vi "Gaussmeter425_BvsTime.vi"() -> ()   [LabVIEW 2014]
uses:
  <vilib>/Platform/TimedLoop/XDataNode/timing_clust.ctl
  <vilib>/Platform/TimedLoop/XDataNode/nitl_modes.ctl
  <vilib>/Platform/TimedLoop/XDataNode/wakeup.ctl
  <instrlib>/Agilent 3446X Series/Public/Data/Read (Single Point).vi
  <instrlib>/Lake Shore 425/Public/Data/Field Data (Single Reading).vi
  <vilib>/Utility/file.llb/Write To Spreadsheet File (DBL).vi
  <vilib>/Platform/TimedLoop/XDataNode/XDataNode.xnode
  <instrlib>/Lake Shore 425/Lake Shore 425.lvlib
  <vilib>/Platform/TimedLoop/XDataNode/XDNodeRunTimeDep.lvlib
  <instrlib>/Agilent 3446X Series/Agilent 3446X Series.lvlib
panel:
  in  "10 A Mode":bool
  out "Output file name":string
  in  "Use multimeter ON / OFF":bool=TRUE
  in  "Comments":string
  in  "Setup":string(combo)
  out "?":dbl(graph)
  in  "VISA resource name MM":refnum<visa-resource-name>="USB0::0x0957::0x1A07::MY53203201::INSTR"
  in  "Measurement Function (10: Voltage DC)":i32(ring)=10 items=["Current DC"=2, "Voltage DC"=10]
  out "Current [A]":dbl
  out "Magnetic Flux [mT]":dbl
  in  "day":dbl
  in  "h":dbl
  in  "min":dbl
  in  "sec":dbl
  out "Time since run start [s]":dbl
  in  "VISA resource name GM":refnum<visa-resource-name>="COM4"
  in  "Measurements per second:":dbl=1.0
  out "?":dbl(graph)
  in  "?":bool
  in  "Serial Configuration":T1={"Baud Rate"=57600, "Parity"=1, "Data Bits"=7, "Stop Bits"=10, "Flow Control"=0} {"Flow Control" items=["None", "XON/XOFF", "RTS/CTS", "XON/XOFF & RTS/CTS", "DTR/DSR", "XON/XOFF & DTR/DSR"]; "Stop Bits" items=["1.0"=10, "1.5"=15, "2.0"=20]; "Data Bits" items=["7"=7, "8"=8]; "Parity" items=["None", "Odd", "Even", "Mark", "Space"]; "Baud Rate" items=["300"=300, "600"=600, "1200"=1200, "2400"=2400, "4800"=4800, "9600"=9600, "19200"=19200, "38400"=38400, "57600"=57600]}
  # "Automatically stop after..."
  # "more than 3 may not work"
  # "Gaussmeter"
  # "Multimeter"
  # "USB0::0x0957: for multimeter"
  # "Voltage DC for Amp"
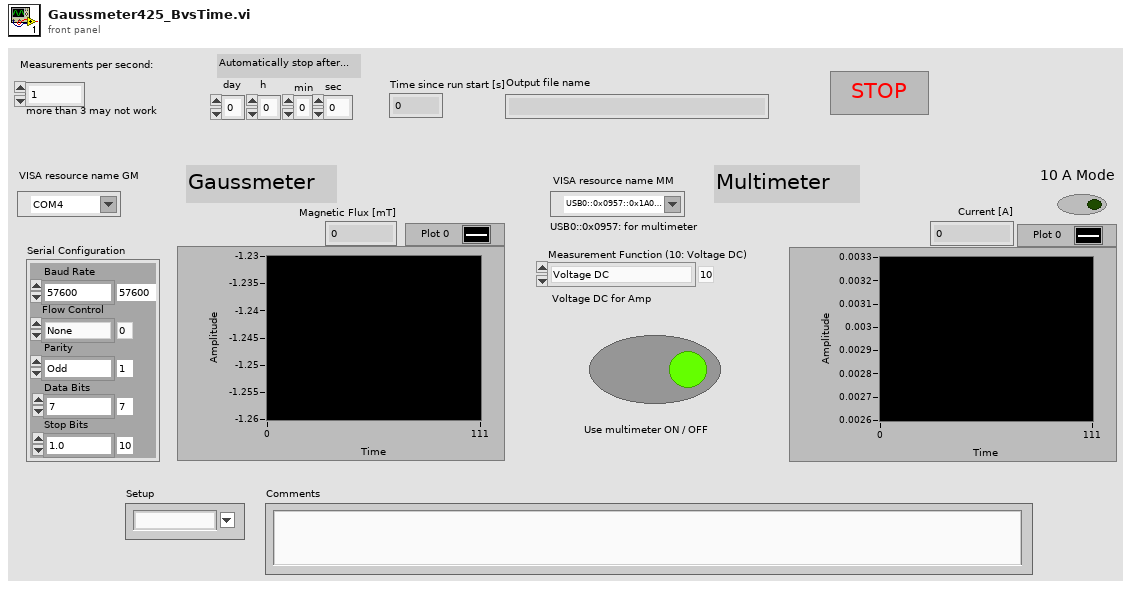
[diagram p1: front panel]
types:
  T1 = cluster{"Baud Rate":u32, "Parity":u16, "Data Bits":u16, "Stop Bits":u16, "Flow Control":u16}
  T2 = typedef "XDNodeRunTimeDep.lvlib/timing_clust.ctl" = cluster{"Expected End [f-1]":u64, "Actual End [f-1]":u64, "Finished Late? [f-1]":bool, "Expected End [i-1]":u64, "Actual End [i-1]":u64, "Finished Late? [i-1]":bool, "Expected Start [i]":u64, "Actual Start [i]":u64, "Expected Start [f]":u64, "Actual Start [f]":u64, "Source Name":string, "Structure Name":string, "Period":i64, "Deadline":i64, "Offset":i64, "Start":i64, "Priority":i32, "Timeout":i32, "Mode":T3, "Wakeup Reason":T4, "Error":errorcluster, "Source Type":string, "Secondary Source Type":string, "Global End Time":u64, "Global Start Time":u64, "Frame Duration":u64, "Iteration Duration":u64, "Assigned CPU":i32, "I/O Scan Engine Mode":u32}
  T3 = typedef "XDNodeRunTimeDep.lvlib/nitl_modes.ctl" = enum32{"No Change", "Process missed periods, maintain original phase", "Discard missed periods, maintain original phase", "Process missed periods, ignore original phase", "Discard missed periods, ignore original phase"}
  T4 = typedef "XDNodeRunTimeDep.lvlib/wakeup.ctl" = enum32{"Normal", "Aborted", "Asynchronous wakeup", "Timing source error", "Timed loop error", "Timeout"}
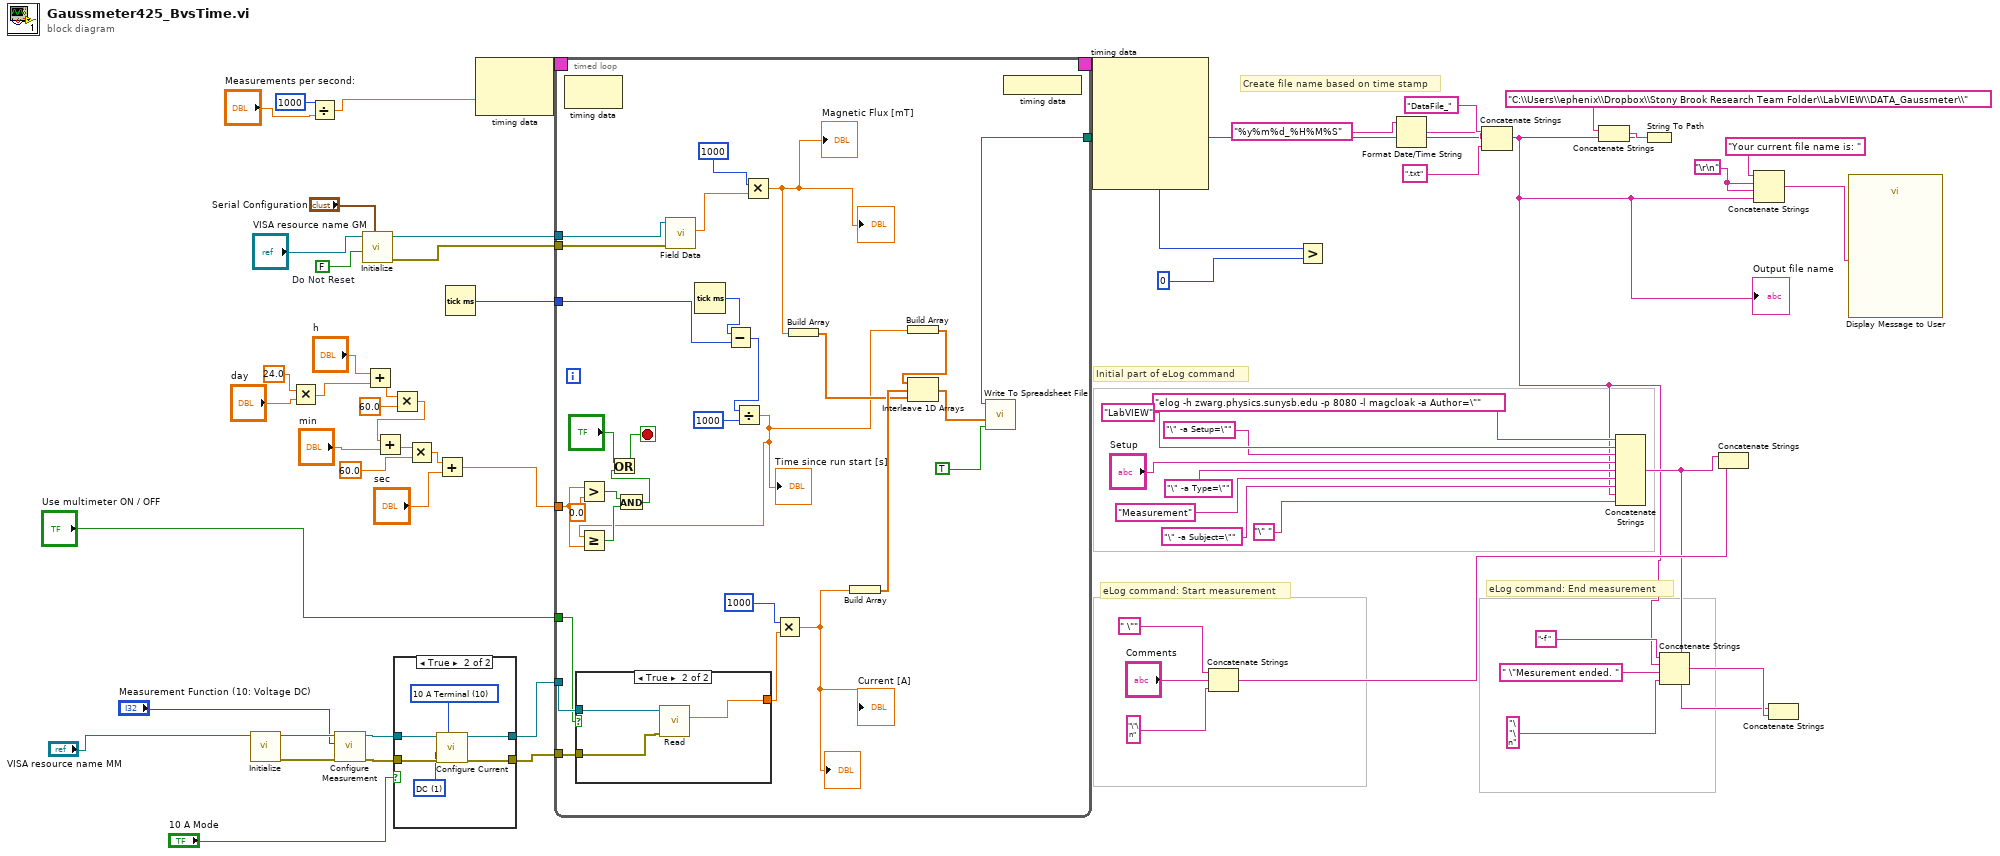
[diagram p0: block diagram]
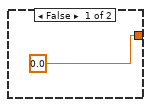
[diagram p3: hidden frame]
diagram:
  w49 = "\r\n"
  w63 = FALSE  # Do Not Reset
  # "eLog command: End measurement"
  # "eLog command: Start measurement"
  # "Initial part of eLog command"
  # "Create file name based on time stamp"
  n1 = call <instrlib>:"Initialize.vi"("VISA resource name"="VISA resource name MM") -> ("error out"=w33:errorcluster, "VISA resource name out"=w34:refnum<visa-resource-name>)  [unwired: 4 in, 5 out]
  n2 = Multiply(x=24.0, y="day") -> (x*y=w44:dbl)
  n3 = Divide(x=1000, y="Measurements per second:") -> (x/y=w47:dbl)
  n4 = call <instrlib>:"Configure Measurement.vi"("error in (no error)"=w33, "Measurement Function (10: Voltage DC)"="Measurement Function (10: Voltage DC)", "VISA resource name"=w34) -> ("error out"=w4:errorcluster, "VISA resource name out"=w2:refnum<visa-resource-name>)  [unwired: 3 in, 4 out]
  n5 = call <instrlib>:"Initialize.vi"("Serial Configuration"="Serial Configuration", "Reset (True)"=w63, "VISA resource name"="VISA resource name GM") -> ("error out"=w60:errorcluster, "VISA resource name out"=w61:refnum<visa-resource-name>)  [unwired: 7 in]
  n6 = Add(x="h", y=w44) -> (x+y=w43:dbl)
  n7 = Multiply(x=w43, y=60.0) -> (x*y=w41:dbl)
  n8 = Add(x=w41, y="min") -> (x+y=w39:dbl)
  n9 = case shown="True" "10 A Mode" {
    tunnel: w4 -> [w65 w72]
    tunnel: [w65 w71] -> w3
    tunnel: w2 -> [w66 w70]
    tunnel: [w66 w69] -> w1
    frame False {
    }
    frame True {
      w67 = 1 items=["AC", "DC"] ("Current Type (0: AC)")
      w68 = 10 items=["3 A Terminal"=3, "10 A Terminal"=10] ("Terminal Type (3: 3 A Terminal)")
      n10 = call <instrlib>:"Configure Current.vi"("Terminal Type (3: 3 A Terminal)"=w68, "error in (no error)"=w72, "Current Type (0: AC)"=w67, "VISA resource name"=w70) -> ("error out"=w71:errorcluster, "VISA resource name out"=w69:refnum<visa-resource-name>)  [unwired: 6 in]
    }
  }
  n11 = Multiply(x=w39, y=60.0) -> (x*y=w37:dbl)
  n12 = Add(x=w37, y="sec") -> (x+y=w35:dbl)
  n13 = Tick Count (ms)() -> (millisecond timer value=w9:u32)
  n14 = node-c288(w47) -> (w59:T2)  [unwired: 1 in]
  n15 = Concatenate Strings(" \"", "Comments", "\"\n") -> (w17:string)
  n16 = Format Date/Time String(time format string (%c)="%y%m%d_%H%M%S") -> (date/time string=w51:string)  [unwired: 2 in]
  n17 = Concatenate Strings("DataFile_", w51, ".txt") -> (w6:string)
  "Output file name" <- w6
  n18 = Concatenate Strings("C:\\Users\\ephenix\\Dropbox\\Stony Brook Research Team Folder\\LabVIEW\\DATA_Gaussmeter\\", w6) -> (w30:string)
  n19 = Concatenate Strings("elog -h zwarg.physics.sunysb.edu -p 8080 -l magcloak -a Author=\"", "LabVIEW", "\" -a Setup=\"", "Setup", "\" -a Type=\"", "Measurement", "\" -a Subject=\"", w6, "\" ") -> (w10:string)
  n20 = String To Path(string=w30) -> (path=w22:path)
  n21 = timed-loop {
    tunnel: w61 -> [w101]
    tunnel: w60 -> [w100]
    timing: w59 -> [_]
    timing-out: [_] -> w58
    tunnel: w35 -> [w91]
    tunnel: w1 -> [w74]
    tunnel: w3 -> [w75]
    tunnel: w22 -> [w84]
    tunnel: w9 -> [w80]
    tunnel: "Use multimeter ON / OFF" -> [w73]
    stop <- w97 stop-if-true
    n22 = node-c288() -> ()  [unwired: 1 in, 1 out]
    n23 = case shown="True" w73 {
      tunnel: [0.0 w105] -> w89
      tunnel: w75 -> [_ w104]
      tunnel: w74 -> [_ w103]
      frame False {
      }
      frame True {
        n24 = call-poly <instrlib>:"Read.vi"("error in (no error)"=w104, "VISA resource name"=w103) -> ("Measurement"=w105:dbl)  [unwired: 2 in, 7 out]
      }
    }
    n25 = Greater?(x=w91, y=0.0) -> (0:w94:bool)
    n26 = call-poly <instrlib>:"Field Data.vi"("error in (no error)"=w100, "VISA resource name"=w101) -> ("Field Reading"=w98:dbl)  [unwired: 7 in, 2 out]
    n27 = Tick Count (ms)() -> (millisecond timer value=w81:u32)
    n28 = Subtract(x=w81, y=w80) -> (x-y=w79:u32)
    n29 = Divide(x=w79, y=u32 1000) -> (x/y=w76:dbl)
    "Time since run start [s]" <- w76
    n30 = Greater Or Equal?(x=w76, y=w91) -> (x >= y?=w93:bool)
    n31 = And(x=w94, y=w93) -> (x .and. y?=w95:bool)
    n32 = Or(x="?", y=w95) -> (x .or. y?=w97:bool)
    n33 = Multiply(x=1000, y=w98) -> (x*y=w90:dbl)
    "?" <- w90
    "Magnetic Flux [mT]" <- w90
    n34 = Multiply(x=1000, y=w89) -> (x*y=w85:dbl)
    "Current [A]" <- w85
    "?" <- w85
    n35 = Build Array(w90) -> (w86:dbl[])
    n36 = Build Array(w85) -> (w87:dbl[])
    n37 = Build Array(w76) -> (w77:dbl[])
    n38 = Interleave 1D Arrays(w77, w87, w86) -> (w83:dbl[])
    n39 = call-poly <vilib>:"Write To Spreadsheet File.vi"("append to file? (new file:F)"=TRUE, "1D data"=w83, "file path (dialog if empty)"=w84) -> ()  [unwired: 5 in, 1 out]
    n40 = node-c288() -> ()  [unwired: 1 out]
  }
  n41 = node-c288(w58) -> (w15:i64)  [unwired: 6 out]
  n42 = Greater?(x=w15, y=0) -> ()  [unwired: 1 out]
  n43 = Concatenate Strings("-f ", w6, " \"Mesurement ended. ", "\"\n") -> (w13:string)
  n44 = Concatenate Strings(w10, w17) -> ()  [unwired: 1 out]
  n45 = Concatenate Strings("Your current file name is: ", w49, w49, w6) -> (w48:string)
  n46 = Concatenate Strings(w10, w13) -> ()  [unwired: 1 out]
  n47 = call "Display Message to User"("Message"=w48) -> ()  [unwired: 9 in, 2 out]
